vi "Write Original.vi"(10 "Sound.lvclass":refnum<class "Sound.lvclass">=refnum, 11 "Sound Modification in":refnum<class "Sound Modification.lvclass">=refnum) -> (3 "Sound Modification out":refnum<class "Sound Modification.lvclass">)   [LabVIEW 2010, in "Sound Modification.lvclass"]
uses:
  Sound Modification.lvclass
  Sound/Sound.lvclass
  Sound Modification.lvclass/Sound Modification.ctl
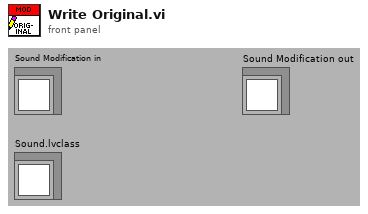
[diagram p1: front panel]
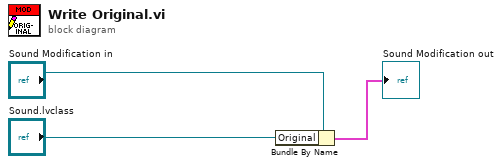
[diagram p0: block diagram]
diagram:
  n1 = Bundle By Name(cluster="Sound Modification in", "Original"="Sound.lvclass") -> (→"Sound Modification out":cluster{})
